vi "Condition Map.vi"(6 "Name Refs.Name VI":refnum<vi>, 8 "error in":errorcluster, 9 "Msg Output All Terminals":i32[](array[numeric]), 10 "Msg All Terminals":i32[](array[numeric])) -> (0 "error out":errorcluster, 1 "Msg Output Terminal Attributes":T1, 2 "Msg Terminal Attributes":T1)   [LabVIEW 2025, in "_Msg Rescript.lvlib" / "_Msg Rescript.lvclass"]
uses:
  _Msg Rescript.lvclass
  Terminal Attributes.ctl
  Attributes.ctl
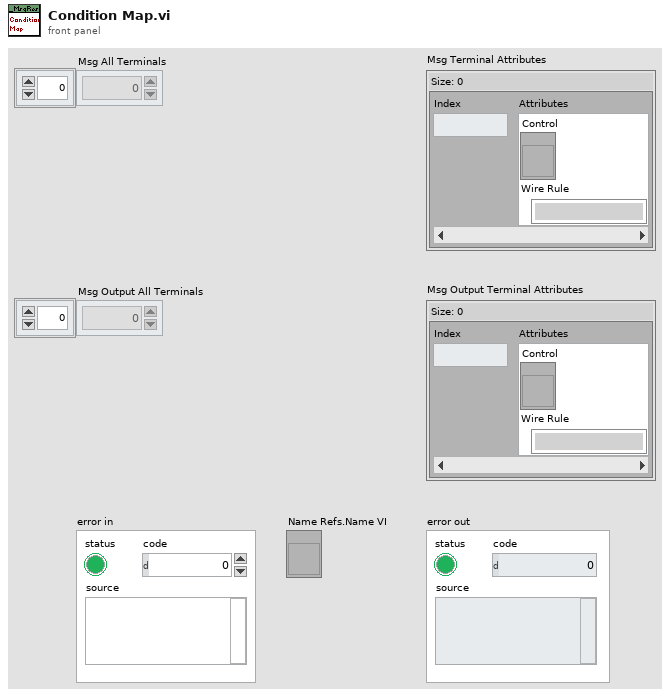
[diagram p1: front panel]
types:
  T1 = typedef "_Msg Rescript.lvlib/_Msg Rescript.lvclass/Terminal Attributes.ctl" = map{i32, T2}
  T2 = typedef "_Msg Rescript.lvlib/_Msg Rescript.lvclass/Attributes.ctl" = cluster{"Control":refnum<vi>, "Wire Rule":enum16{"Invalid Wire Rule", "Required", "Recommended", "Optional", "Dynamic Dispatch"}}
  T3 = enum16{"Invalid Wire Rule", "Required", "Recommended", "Optional", "Dynamic Dispatch"}[]
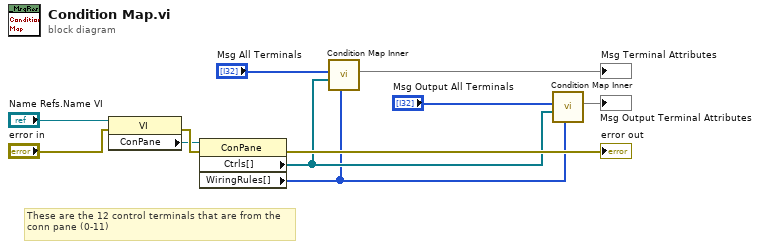
[diagram p0: block diagram]
diagram:
  # "These are the 12 control terminals that are from the conn pane (0-11)"
  n1 = property class="VI"(reference="Name Refs.Name VI", error in="error in") -> (error out=w10:errorcluster, "ConPane"=w9:refnum<vi>)  [unwired: 1 out]
  n2 = property class="ConPane"(reference=w9, error in=w10) -> (error out=→"error out":errorcluster, "Ctrls[]"=w2:refnum<vi>[], "WiringRules[]"=w1:T3)  [unwired: 1 out]
  n3 = call "Condition Map Inner.vi"("WiringRules[]"=w1, "Controls[]"=w2, "All Terminals"="Msg All Terminals") -> ("Terminal Attributes"=→"Msg Terminal Attributes":T1)  [unwired: 8 in]
  n4 = call "Condition Map Inner.vi"("WiringRules[]"=w1, "Controls[]"=w2, "All Terminals"="Msg Output All Terminals") -> ("Terminal Attributes"=→"Msg Output Terminal Attributes":T1)  [unwired: 8 in]
